vi "Main.vi"(11 "Module Admin":refnum<class "Delacor_lib_QMH_Module Admin.lvclass">) -> ()   [LabVIEW 2020, in "Logger.lvlib"]
doc: "This template is based off of the Queued Message Handler design pattern and the Queued Message Handler project template that ships with LabVIEW.\n\nThe main difference is that the queue is private to this module and communication between modules is performed via Broadcast and Request events.\n\nRequest events are wrapped in public API methods and are handled in the Event Handling Loop (EHL) of this VI. Any module can register for Broadcast events sent by this module. The EHL generates messages based on user interface actions.\n\nThe Message Handling Loop (MHL) processes messages generated by the EHL, or by other messages. The messages are string values, so new messages can be added easily to the Message Cases case structure in the MHL. Each message cluster can also provide an optional value for Message Data, which is a variant that can be converted to whatever message-specific data is required.\n_____\nBased on DQMH Project Template 4.0.0.47.\n_____\nBased on DQMH Project Template 7.0.1.1316."
uses:
  Logger.lvlib
  Module Data--cluster.ctl
  <vilib>/Delacor/Delacor QMH/Libraries/Message Queue_class/Delacor_lib_QMH_Message Queue.lvclass
  <vilib>/Delacor/Delacor QMH/Libraries/Message Queue_class/Delacor_lib_QMH_Enqueue Message (Single).vi
  <vilib>/Delacor/Delacor QMH/Libraries/Module Admin_class/Delacor_lib_QMH_Module Admin.lvclass
  Stop Argument--cluster.ctl
  <vilib>/Utility/miscctls.llb/LVPointTypeDef.ctl
  Stop Logging Argument--cluster.ctl
  Settings Editor/Settings Editor.lvlib
  Log Data Argument--cluster.ctl
  CML Shared/Signal Type--enum.ctl
  CML Shared/CML Shared.lvlib
  Settings Editor/Settings--cluster.ctl
  CML Shared/Calibration Values--cluster.ctl
  Initialize File (Reply Payload)--cluster.ctl
  Initialize File Argument--cluster.ctl
  Settings Editor/Update Application Settings (Reply Payload)--cluster.ctl
  <vilib>/Peloton/Peloton Config/DCFG Framework/Peloton_lib_DCFG Framework.lvlib
  Configuration/Configuration.lvclass
  Configuration/Configuration--cluster.ctl
  <vilib>/Peloton/Peloton Config/DCFG Framework/Configuration_class/Configuration.lvclass
panel:
  out "Settings":T1
  out "error out":errorcluster
  # "This is a headless module. Show its panel to confirm that the Settings are updated correctly and other debugging tasks. Use the Settings Editor to change the settings for this module."
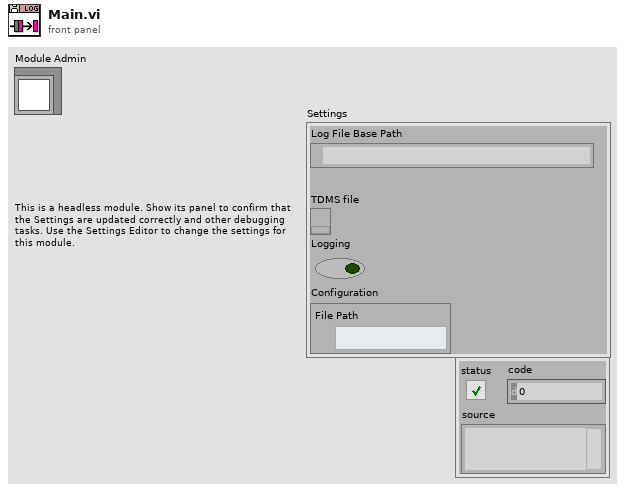
[diagram p1: front panel]
types:
  T1 = typedef "Logger.lvlib/Module Data--cluster.ctl" = cluster{"Log File Base Path":path, "TDMS file":refnum<k34>, "Logging":bool, "Configuration":T2}
  T2 = typedef "Logger.lvlib/Configuration.lvclass/Configuration--cluster.ctl" = cluster{"File Path":path}
  T3 = typedef "Settings Editor.lvlib/Broadcast Events--cluster.ctl" = cluster{"Module Did Init":refnum<user-event>, "Status Updated":refnum<user-event>, "Error Reported":refnum<user-event>, "Module Did Stop":refnum<user-event>, "Update Module Execution Status":refnum<user-event>, "Application Settings Updated":refnum<user-event>}
  T4 = typedef "Logger.lvlib/Request Events--cluster.ctl" = cluster{"Stop Module":refnum<user-event>, "Show Panel":refnum<user-event>, "Hide Panel":refnum<user-event>, "Get Module Execution Status":refnum<user-event>, "Show Diagram":refnum<user-event>, "Stop Logging":refnum<user-event>, "Log Data":refnum<user-event>, "Initialize File":refnum<user-event>}
  T5 = typedef "Peloton_lib_DCFG Framework.lvlib/Broadcast Events--cluster.ctl" = cluster{"Module Did Init":refnum<user-event>, "Status Updated":refnum<user-event>, "Error Reported":refnum<user-event>, "Module Did Stop":refnum<user-event>, "Update Module Execution Status":refnum<user-event>, "View Changed":refnum<user-event>, "Main Window Closed":refnum<user-event>, "Configuration Committed":refnum<user-event>, "Configuration Canceled":refnum<user-event>, "Views List Updated":refnum<user-event>, "Config Folder Path Updated":refnum<user-event>}
  T6 = enum32{"invalid lock state", "Not Locked", "Locked (No Password)", "Password-protected"}
  T7 = typedef "Logger.lvlib/Stop Argument--cluster.ctl" = cluster{"Origin":string, "Exit via Stop Module Req?":bool, "Wait for Module to stop?":bool}
  T8 = typedef "Logger.lvlib/Initialize File Argument--cluster.ctl" = cluster{"Wait Notifier":refnum<notifier>, "wait for reply":bool}
  T9 = typedef "Logger.lvlib/Log Data Argument--cluster.ctl" = cluster{"Waveforms":waveform(dbl)[]}
  T10 = typedef "Logger.lvlib/Stop Logging Argument--cluster.ctl" = cluster{"Boolean":bool}
  T11 = typedef "Settings Editor.lvlib/Update Application Settings (Reply Payload)--cluster.ctl" = cluster{"Settings":T12, "error":errorcluster}
  T12 = typedef "Settings Editor.lvlib/Settings--cluster.ctl" = cluster{"Signal Type":T13, "Calibration Array":T14[], "Log File Base Path":path}
  T13 = typedef "CML Shared.lvlib/Signal Type--enum.ctl" = enum16{"Sine Wave", "Square with Noise"}
  T14 = typedef "CML Shared.lvlib/Calibration Values--cluster.ctl" = cluster{"Slope":dbl, "Offset":dbl}
  T15 = typedef "LVPointTypeDef.ctl" = cluster{"Horizontal":i16, "Vertical":i16}
  T16 = enum32{"Invalid", "Standard", "Closed", "Hidden", "Minimized", "Maximized"}
  T17 = typedef "Logger.lvlib/Initialize File (Reply Payload)--cluster.ctl" = cluster{"File Path":path, "error":errorcluster}
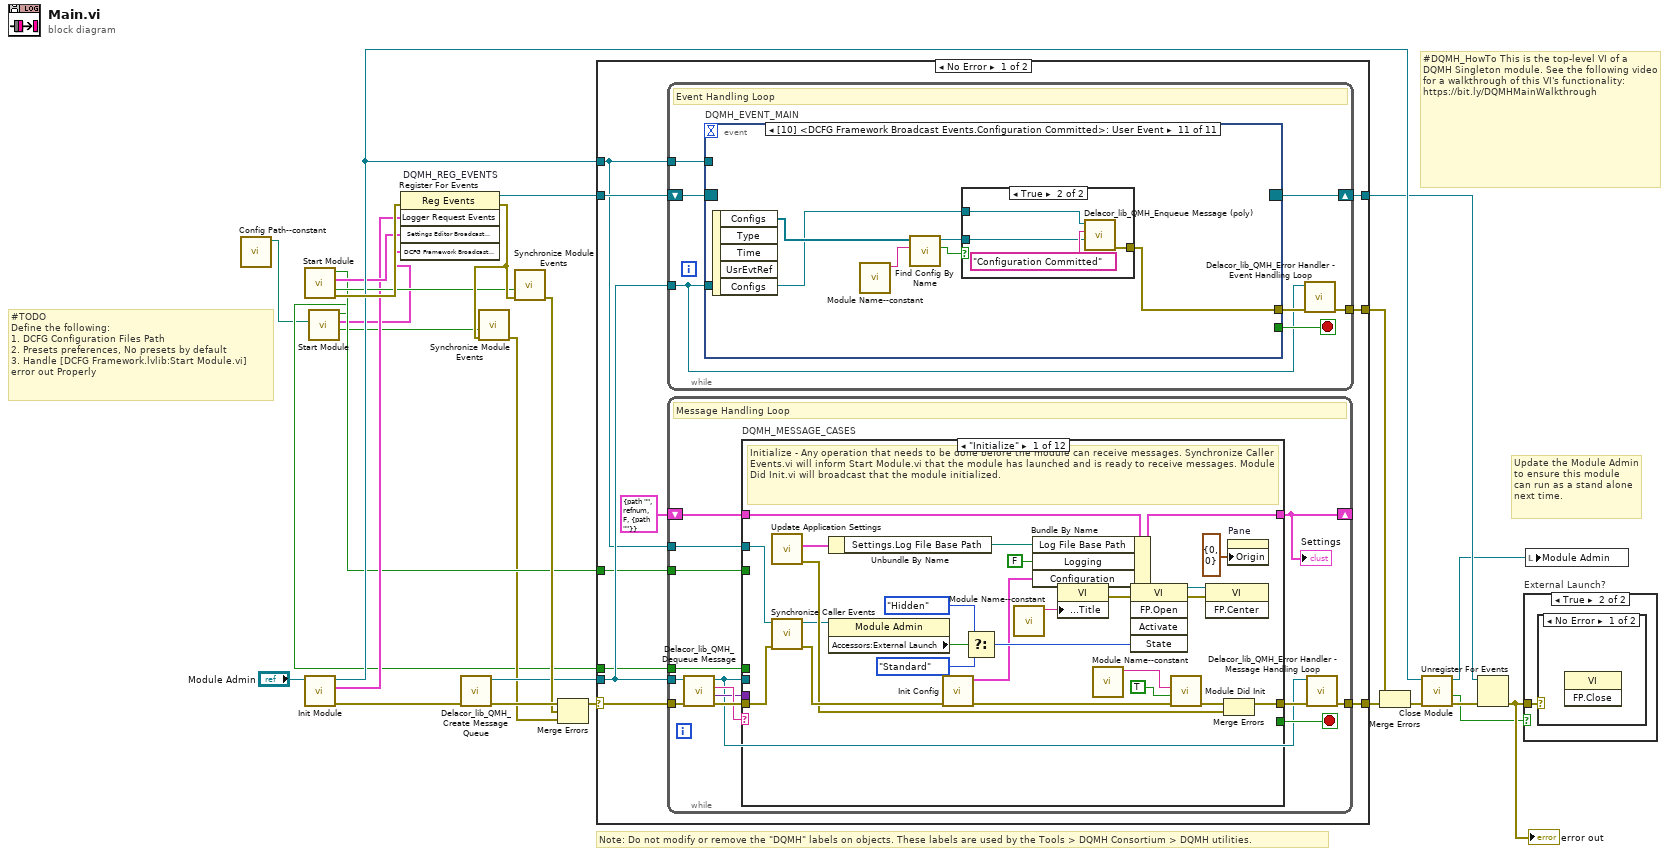
[diagram p0: block diagram]
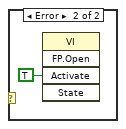
[diagram p3: hidden frame]
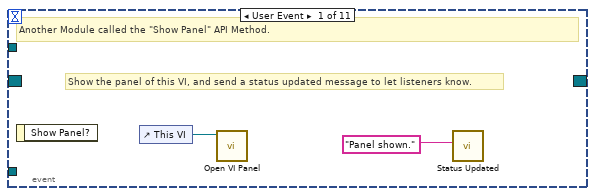
[diagram p4: hidden frame]
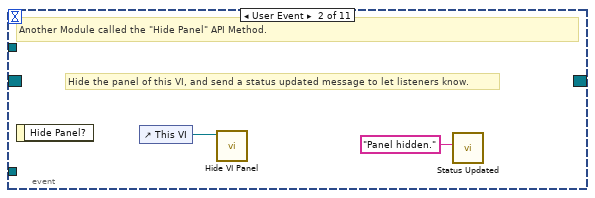
[diagram p5: hidden frame]
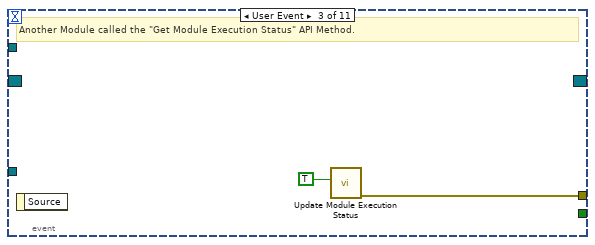
[diagram p6: hidden frame]
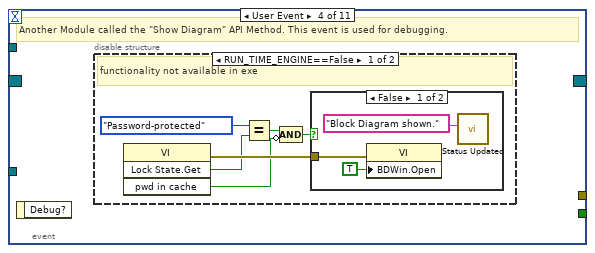
[diagram p7: hidden frame]
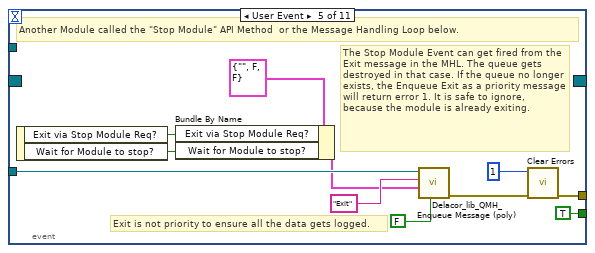
[diagram p10: hidden frame]
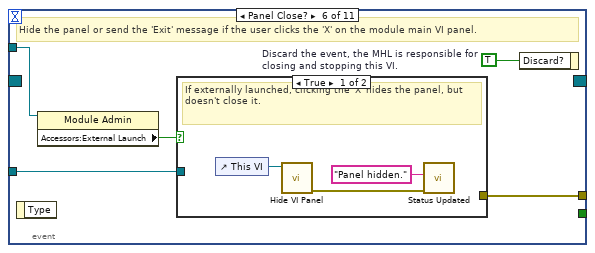
[diagram p11: hidden frame]
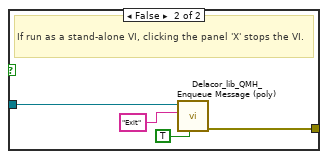
[diagram p12: hidden frame]
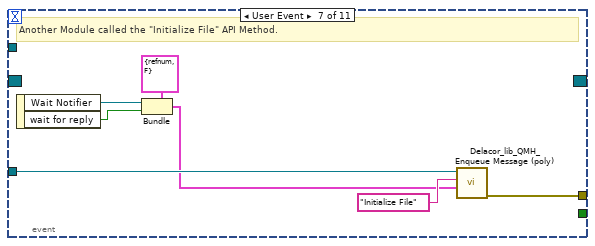
[diagram p13: hidden frame]
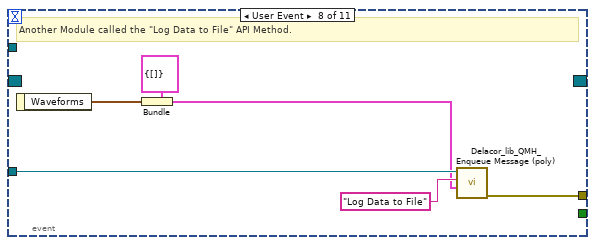
[diagram p14: hidden frame]
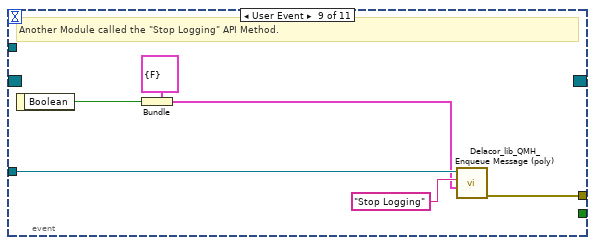
[diagram p15: hidden frame]
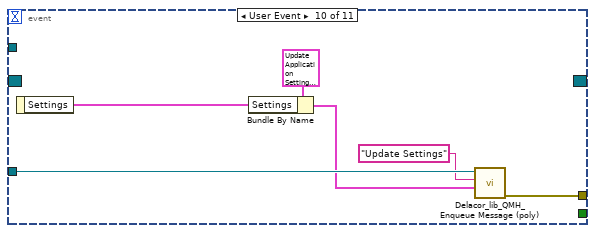
[diagram p16: hidden frame]
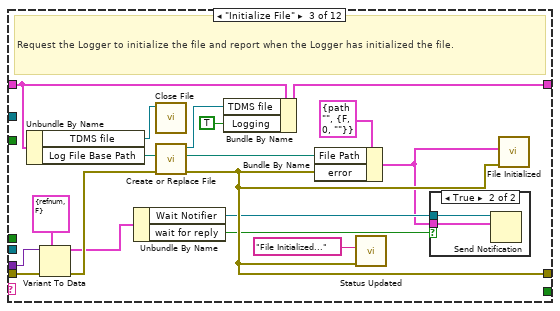
[diagram p19: hidden frame]
diagram:
  # "#TODO\nDefine the following:\n1. DCFG Configuration Files Path\n2. Presets preferences, No presets by default\n3. Handle [DCFG Framework.lvlib:Start Module.vi]\nerror out Properly"
  # "#DQMH_HowTo This is the top-level VI of a DQMH Singleton module. See the following video for a walkthrough of this VI's functionality: https://bit.ly/DQMHMainWalkthrough"
  # "Note: Do not modify or remove the \"DQMH\" labels on objects. These labels are used by the Tools > DQMH Consortium > DQMH utilities."
  # "Update the Module Admin to ensure this module can run as a stand alone next time."
  n1 = call "Config Path--constant.vi"() -> ("File Path"=w1:path)  [unwired: 11 in]
  n2 = call <vilib>:"Start Module.vi"() -> ("error out"=w19:errorcluster, "Wait for Event Sync?"=w9:bool, "Settings Editor Broadcast Events"=w8:T3, "Module Was Already Running?"=w6:bool)  [unwired: 8 in]
  n3 = call "Init Module.vi"("Singleton Module Admin in"="Module Admin") -> ("error out"=w26:errorcluster, "Logger Request Events"=w7:T4, "Singleton Module Admin out"=w16:refnum<class "Delacor_lib_QMH_Module Admin.lvclass">)  [unwired: 8 in]
  n4 = call <vilib>:"Start Module.vi"("Config Folder"=w1) -> ("Wait for Event Sync?"=w4:bool, "DCFG Framework Broadcast Events"=w5:T5, "Module Was Already Running?"=w2:bool)  [unwired: 7 in, 1 out]
  n5 = register-events "DQMH_REG_EVENTS"(error in=w19, w7, w8, w5) -> (reference out=w14:refnum<event-registration>, error out=w18:errorcluster)  [unwired: 1 in]
  n6 = call <vilib>:"Delacor_lib_QMH_Create Message Queue.vi"("error in"=w26) -> ("error out"=w21:errorcluster, "Message Queue"=w13:refnum<class "Delacor_lib_QMH_Message Queue.lvclass">)  [unwired: 9 in]
  n7 = call <vilib>:"Synchronize Module Events.vi"("error in (no error)"=w18, "Wait for Event Sync?"=w4) -> ("error out"=w3:errorcluster)  [unwired: 9 in]
  n8 = call <vilib>:"Synchronize Module Events.vi"("error in"=w18, "Wait for Event Sync?"=w9) -> ("error out"=w17:errorcluster)  [unwired: 9 in]
  n9 = Merge Errors(w21, w17, w3) -> (w20:errorcluster)
  n10 = case shown="No Error" w20 {
    selector: w20 -> [w35 w287]
    tunnel: [w37 w286] -> w27
    tunnel: [w34 w285] -> w15
    tunnel: w14 -> [w32 w285]
    tunnel: w13 -> [w31 w279]
    tunnel: [w36 _] -> w24
    tunnel: w16 -> [w30 w281]
    tunnel: w6 -> [w29 w280]
    tunnel: w2 -> [w28 w278]
    frame No Error {
      n11 = while {
        tunnel: w31 -> [w38]
        shift-right: [w41] -> w34
        shift-left: w32 -> [w42]
        tunnel: [w43] -> w36
        tunnel: w30 -> [w39]
        stop <- w40 stop-if-true
        # "Event Handling Loop"
        n12 = event "DQMH_EVENT_MAIN" shown="[10] <DCFG Framework Broadcast Events.Configuration Committed>: User Event" {
          selector: w42 -> [_ _ _ _ _ _ _ _ _ _ _]
          dyn-events: [_ _ _ _ _ _ _ _ _ _ _] -> w41
          timeout: _ -> [_ _ _ _ _ _ _ _ _ _ _]
          tunnel: [_ _ _ _ TRUE ("Discard?") _ _ _ _ _ _] -> w40
          tunnel: w38 -> [_ _ _ _ w66 w73 w88 w94 w100 w106 w111]
          tunnel: [_ _ w50 _ w69 w75 w89 w95 w101 w107 w113] -> w44
          tunnel: w39 -> [_ _ _ _ _ w72 _ _ _ _ _]
          event User Event {
            # "Show the panel of this VI, and send a status updated message to let listeners know."
            # "Another Module called the \"Show Panel\" API Method."
            n13 = event-data() -> ()  [unwired: 1 in, 1 out]
            n14 = control-ref of="This VI"() -> (w46:refnum<vi>)
            n15 = call "Open VI Panel.vi"("VI"=w46) -> ()  [unwired: 10 in, 1 out]
            n16 = call "Status Updated.vi"("Status"="Panel shown." ("format string")) -> ()  [unwired: 10 in, 1 out]
          }
          event User Event {
            # "Hide the panel of this VI, and send a status updated message to let listeners know."
            # "Another Module called the \"Hide Panel\" API Method."
            n17 = event-data() -> ()  [unwired: 1 in, 1 out]
            n18 = control-ref of="This VI"() -> (w48:refnum<vi>)
            n19 = call "Hide VI Panel.vi"("VI"=w48) -> ()  [unwired: 10 in, 1 out]
            n20 = call "Status Updated.vi"("Status"="Panel hidden." ("format string")) -> ()  [unwired: 10 in, 1 out]
          }
          event User Event {
            # "Another Module called the \"Get Module Execution Status\" API Method."
            n21 = event-data() -> ()  [unwired: 1 in, 1 out]
            n22 = call "Update Module Execution Status.vi"("Running?"=TRUE) -> ("error out"=w50:errorcluster)  [unwired: 10 in]
          }
          event User Event {
            # "Another Module called the \"Show Diagram\" API Method. This event is used for debugging."
            n23 = event-data() -> ()  [unwired: 1 in, 1 out]
            n24 = disable-structure shown="RUN_TIME_ENGINE==False" {
              frame condition #0 (active) {
                # "functionality not available in exe"
                n25 = invoke on="Invoke Node" class="VI" method="Lock State.Get"() -> (error out=w56:errorcluster, "Get Lock State"=w55:T6, "pwd in cache"=w52:bool)  [unwired: 4 in, 1 out]
                n26 = Equal?(x=T6."Password-protected", y=w55) -> (x = y?=w53:bool)
                n27 = Compound Arithmetic op=AND(w53, invert w52) -> (w51:bool)
                n28 = case shown="False" w51 {
                  tunnel: w56 -> [w59 _]
                  frame False {
                    n29 = property on="Property Node" class="VI"(error in=w59, "BDWin.Open"=TRUE ("Block Diagram Window:Open")) -> ()  [unwired: 1 in, 2 out]
                    n30 = call "Status Updated.vi"("Status"="Block Diagram shown." ("format string")) -> ()  [unwired: 10 in, 1 out]
                  }
                  frame True {
                    # "Password-protected VI, and the password is not in the cache. Do not show the diagram."
                  }
                }
              }
              frame condition #1 {
              }
            }
          }
          event User Event {
            # "Exit is not priority to ensure all the data gets logged."
            # "The Stop Module Event can get fired from the Exit message in the MHL. The queue gets destroyed in that case. If the queue no longer exists, the Enqueue Exit as a priority message will return error 1. It is safe to ignore, because the module is already exiting."
            # "Another Module called the \"Stop Module\" API Method  or the Message Handling Loop below."
            n31 = event-data() -> ("Exit via Stop Module Req?"=w62:bool, "Wait for Module to stop?"=w61:bool)  [unwired: 1 in]
            n32 = Bundle By Name(cluster=T7 {"Origin"="", "Exit via Stop Module Req?"=FALSE, "Wait for Module to stop?"=FALSE} ("Stop Argument"), "Exit via Stop Module Req?"=w62, "Wait for Module to stop?"=w61) -> (w60:T7)
            n33 = call-poly <vilib>:"Delacor_lib_QMH_Enqueue Message (poly).vi"("Priority Message? (F)"=FALSE, "Message Data"=w60, "Message"="Exit", "Message Queue in"=w66) -> ("error out"=w70:errorcluster)  [unwired: 6 in, 1 out]
            n34 = call <vilib>:"Clear Errors.vi"("error in (no error)"=w70, "specific error code to clear (0: all)"=1) -> ("error out"=w69:errorcluster)  [unwired: 4 in, 1 out]
          }
          event Panel Close? {
            w74 = TRUE  # Discard the event, the MHL is responsible for closing and stopping this VI.
            # "Hide the panel or send the 'Exit' message if the user clicks the 'X' on the module main VI panel."
            n35 = event-data() -> ()  [unwired: 1 in, 1 out]
            n36 = property on="Property Node" class="Module Admin"(reference=w72) -> ("Accessors:External Launch"=w71:bool)  [unwired: 1 in, 2 out]
            n37 = case shown="True" w71 {
              tunnel: w73 -> [_ w81]
              tunnel: [_ w82] -> w75
              frame True {
                # "If externally launched, clicking the 'X' hides the panel, but doesn't close it."
                n38 = control-ref of="This VI"() -> (w78:refnum<vi>)
                n39 = call "Hide VI Panel.vi"("VI"=w78) -> ("error out"=w76:errorcluster)  [unwired: 10 in]
                n40 = call "Status Updated.vi"("error in"=w76, "Status"="Panel hidden." ("format string")) -> ()  [unwired: 9 in, 1 out]
              }
              frame False {
                # "If run as a stand-alone VI, clicking the panel 'X' stops the VI."
                n41 = call-poly <vilib>:"Delacor_lib_QMH_Enqueue Message (poly).vi"("Priority Message? (F)"=TRUE, "Message"="Exit", "Message Queue in"=w81) -> ("error out"=w82:errorcluster)  [unwired: 7 in, 1 out]
              }
            }
            n42 = event-data ("Event Filter Node")("Discard?"=w74) -> ()  [unwired: 1 in, 1 out]
          }
          event User Event {
            # "Another Module called the \"Initialize File\" API Method."
            n43 = event-data() -> ("Wait Notifier"=w84:refnum<notifier>, "wait for reply"=w83:bool)  [unwired: 1 in]
            n44 = Bundle(cluster=T8 {"Wait Notifier"=refnum, "wait for reply"=FALSE} ("Initialize File Argument"), "Wait Notifier"=w84, "wait for reply"=w83) -> (w85:T8)
            n45 = call-poly <vilib>:"Delacor_lib_QMH_Enqueue Message (poly).vi"("Message Data"=w85, "Message"="Initialize File", "Message Queue in"=w88) -> ("error out"=w89:errorcluster)  [unwired: 7 in, 1 out]
          }
          event User Event {
            # "Another Module called the \"Log Data to File\" API Method."
            n46 = event-data() -> ("Waveforms"=w90:waveform(dbl)[])  [unwired: 1 in]
            n47 = Bundle(cluster=T9 {"Waveforms"=[]} ("Log Data to File Argument"), "Waveforms"=w90) -> (w91:T9)
            n48 = call-poly <vilib>:"Delacor_lib_QMH_Enqueue Message (poly).vi"("Message Data"=w91, "Message"="Log Data to File", "Message Queue in"=w94) -> ("error out"=w95:errorcluster)  [unwired: 7 in, 1 out]
          }
          event User Event {
            # "Another Module called the \"Stop Logging\" API Method."
            n49 = event-data() -> ("Boolean"=w96:bool)  [unwired: 1 in]
            n50 = Bundle(cluster=T10 {"Boolean"=FALSE} ("Stop Logging Argument"), "Boolean"=w96) -> (w97:T10)
            n51 = call-poly <vilib>:"Delacor_lib_QMH_Enqueue Message (poly).vi"("Message Data"=w97, "Message"="Stop Logging", "Message Queue in"=w100) -> ("error out"=w101:errorcluster)  [unwired: 7 in, 1 out]
          }
          event User Event {
            n52 = event-data() -> ("Settings"=w103:T12)  [unwired: 1 in]
            n53 = Bundle By Name(cluster=T11 {"Settings"={"Signal Type"=enum."Sine Wave", "Calibration Array"=[], "Log File Base Path"=path ""}, "error"={"status"=FALSE, "code"=0, "source"=""}} ("Settings Updated Argument"), "Settings"=w103) -> (w102:T11)
            n54 = call-poly <vilib>:"Delacor_lib_QMH_Enqueue Message (poly).vi"("Message Data"=w102, "Message"="Update Settings", "Message Queue in"=w106) -> ("error out"=w107:errorcluster)  [unwired: 7 in, 1 out]
          }
          event User Event {
            n55 = event-data() -> ("Configs"=w112:refnum<class "Configuration.lvclass">[])  [unwired: 1 in, 4 out]
            n56 = call "Module Name--constant.vi"() -> ("Module Name"=w110:string)  [unwired: 11 in]
            n57 = call <vilib>:"Find Config By Name.vi"("Config Name"=w110, "All Config Classes"=w112) -> ("Found"=w109:bool, "Configuration"=w108:refnum<class "Configuration.lvclass">)  [unwired: 6 in, 2 out]
            n58 = case shown="True" w109 {
              tunnel: w111 -> [_ w116]
              tunnel: [_ w117] -> w113
              tunnel: w108 -> [_ w114]
              frame False {
              }
              frame True {
                n59 = call-poly <vilib>:"Delacor_lib_QMH_Enqueue Message (poly).vi"("Message Data"=w114, "Message"="Configuration Committed", "Message Queue in"=w116) -> ("error out"=w117:errorcluster)  [unwired: 7 in, 1 out]
              }
            }
          }
        }
        n60 = call-dynamic "Delacor_lib_QMH_Error Handler - Event Handling Loop.vi"("error in"=w44, "Message Queue in"=w38) -> ("dup error in"=w43:errorcluster)  [unwired: 8 in, 1 out]
      }
      n61 = while {
        tunnel: w31 -> [w122]
        shift-right: [w126] -> _
        shift-left: T1 {"Log File Base Path"=path "", "TDMS file"=refnum, "Logging"=FALSE, "Configuration"={"File Path"=path ""}} ("Data Cluster") -> [w127]
        tunnel: w35 -> [w130]
        tunnel: [w128] -> w37
        tunnel: w30 -> [w120]
        tunnel: w29 -> [w119]
        tunnel: w28 -> [w118]
        stop <- w125 stop-if-true
        # "Message Handling Loop"
        n62 = call-dynamic "Delacor_lib_QMH_Dequeue Message.vi"("error in"=w130, "Message Queue in"=w122) -> ("error out"=w129:errorcluster, "Message Data"=w123:variant, "Message"=w124:string, "Message Queue out"=w121:refnum<class "Delacor_lib_QMH_Message Queue.lvclass">)  [unwired: 6 in]
        n63 = case "DQMH_MESSAGE_CASES" shown="\"Initialize\"" w124 {
          selector: w124 -> [_ _ _ _ _ _ _ _ _ _ w265 _]
          tunnel: w121 -> [_ _ _ _ _ _ _ _ w225 w251 _ _]
          tunnel: w129 -> [w155 w159 w176 w188 w201 w211 w219 w221 w232 w257 w268 w277]
          tunnel: [w152 w159 w177 w187 w200 w209 w218 w221 w228 w252 w269 w274] -> w131
          tunnel: w127 -> [w142 w158 w165 w184 w199 w204 w217 w220 w227 w243 w266 w276]
          tunnel: [w136 w158 w164 w181 w197 w204 w217 w220 w227 w243 w266 w275] -> w126
          tunnel: [_ _ _ _ _ _ _ _ _ w250 _ _] -> w125
          tunnel: w123 -> [_ _ w174 w186 w198 w208 _ _ w226 w249 _ w273]
          tunnel: w120 -> [w143 _ _ _ _ _ _ _ w224 w244 _ _]
          tunnel: w119 -> [_ _ _ _ _ _ _ _ _ w241 _ _]
          tunnel: w118 -> [_ _ _ _ _ _ _ _ _ w239 _ _]
          frame "Initialize" {
            # "Initialize - Any operation that needs to be done before the module can receive messages. Synchronize Caller Events.vi will inform Start Module.vi that the module has launched and is ready to receive messages. Module Did Init.vi will broadcast that the module initialized."
            n64 = call "Update Application Settings.vi"() -> ("error out"=w151:errorcluster, "Reply Payload"=w137:T11)  [unwired: 9 in, 1 out]
            n65 = call "Synchronize Caller Events.vi"("error in"=w155, "Singleton Module Admin in"=w143) -> ("error out"=w154:errorcluster, "Singleton Module Admin out"=w139:refnum<class "Delacor_lib_QMH_Module Admin.lvclass">)  [unwired: 8 in]
            n66 = Unbundle By Name(w137) -> ("Settings.Log File Base Path"=w135:path)
            n67 = property on="Property Node" class="Module Admin"(reference=w139) -> ("Accessors:External Launch"=w147:bool)  [unwired: 1 in, 2 out]
            n68 = call "Init Config.vi"("error in"=w154) -> ("error out"=w133:errorcluster, "Configuration"=w132:T2)  [unwired: 9 in]
            n69 = Select(t=T16."Hidden" ("State"), s=w147, f=T16."Standard" ("State")) -> (s? t:f=w144:T16)
            n70 = call "Module Name--constant.vi"() -> ("Module Name"=w150:string)  [unwired: 11 in]
            n71 = Bundle By Name(cluster=w142, "Log File Base Path"=w135, "Logging"=FALSE, "Configuration"=w132) -> (w136:T1)
            n72 = property on="Property Node" class="VI"("Front Panel.Title"=w150) -> (reference out=w149:refnum<vi>, error out=w157:errorcluster)  [unwired: 2 in]
            n73 = call "Module Name--constant.vi"() -> ("Module Name"=w140:string)  [unwired: 11 in]
            n74 = invoke on="Invoke Node" class="VI" method="FP.Open"(reference=w149, error in=w157, "State"=w144) -> (reference out=w148:refnum<vi>, error out=w156:errorcluster)  [unwired: 2 in, 3 out]
            n75 = call "Module Did Init.vi"("error in"=w133, "Initialized?"=TRUE, "Origin"=w140) -> ("error out"=w153:errorcluster)  [unwired: 8 in]
            n76 = invoke on="Invoke Node" class="VI" method="FP.Center"(reference=w148, error in=w156) -> ()  [unwired: 1 in, 3 out]
            n77 = Merge Errors(w153, w151) -> (w152:errorcluster)
            n78 = property on="Pane" class="Pane"("Origin"=T15 {"Horizontal"=0, "Vertical"=0}) -> ()  [unwired: 2 in, 2 out]
          }
          frame "---Module Specific---" {
            # "Separator -- The following cases handle messages specific to this Module."
          }
          frame "Initialize File" {
            # "Request the Logger to initialize the file and report when the Logger has initialized the file."
            n79 = Unbundle By Name(w165) -> ("TDMS file"=w160:refnum<k34>, "Log File Base Path"=w167:path)
            n80 = Variant To Data(error in=w176, type=T8 {"Wait Notifier"=refnum, "wait for reply"=FALSE} ("Initialize File Argument"), Variant=w174) -> (data=w172:T8, error out=w175:errorcluster)
            n81 = Unbundle By Name(w172) -> ("Wait Notifier"=w171:refnum<notifier>, "wait for reply"=w170:bool)
            n82 = call "Close File.vi"("Refnum out"=w160) -> ()  [unwired: 10 in, 1 out]
            n83 = call "Create or Replace File.vi"("error in"=w175, "Log File Base Path"=w167) -> ("error out"=w177:errorcluster, "File Path"=w163:path, "Refnum out"=w166:refnum<k34>)  [unwired: 7 in]
            n84 = Bundle By Name(cluster=w165, "TDMS file"=w166, "Logging"=TRUE) -> (w164:T1)
            n85 = Bundle By Name(cluster=T17 {"File Path"=path "", "error"={"status"=FALSE, "code"=0, "source"=""}} ("Initialize File (Reply Payload)"), "File Path"=w163, "error"=w177) -> (w168:T17)
            n86 = call "Status Updated.vi"("error in"=w177, "Status"="File Initialized...") -> ()  [unwired: 9 in, 1 out]
            n87 = case shown="True" w170 {
              tunnel: w171 -> [_ w179]
              tunnel: w168 -> [_ w178]
              frame False {
              }
              frame True {
                n88 = Send Notification(notification=w178, notifier=w179) -> ()  [unwired: 1 in, 2 out]
              }
            }
            n89 = call "File Initialized.vi"("error in"=w177, "Reply Payload"=w168) -> ()  [unwired: 9 in, 1 out]
          }
          frame "Stop Logging" {
            # "Requests Logger module to stop logging and the module broadcasts when the logging has stopped."
            n90 = Variant To Data(error in=w188, type=T10 {"Boolean"=FALSE} ("Stop Logging Argument"), Variant=w186) -> (error out=w187:errorcluster)  [unwired: 1 out]
            n91 = Unbundle By Name(w184) -> ("Logging"=w183:bool, "TDMS file"=w182:refnum<k34>)
            n92 = case shown="True" w183 {
              tunnel: w187 -> [_ w192]
              tunnel: w182 -> [_ w189]
              frame False {
                # "We were not logging, so this is a no-op."
              }
              frame True {
                n93 = call "Close File.vi"("Refnum out"=w189) -> ()  [unwired: 10 in, 1 out]
                n94 = call "Logging Stopped.vi"("error in"=w192) -> ("error out"=w191:errorcluster)  [unwired: 10 in]
                n95 = call "Status Updated.vi"("error in"=w191, "Status"="Logging Stopped...") -> ()  [unwired: 9 in, 1 out]
              }
            }
            n96 = Bundle By Name(cluster=w184, "Logging"=FALSE) -> (w181:T1)
          }
          frame "Update Settings" {
            n97 = Variant To Data(error in=w201, type=T11 {"Settings"={"Signal Type"=enum."Sine Wave", "Calibration Array"=[], "Log File Base Path"=path ""}, "error"={"status"=FALSE, "code"=0, "source"=""}} ("Settings Updated Argument"), Variant=w198) -> (data=w196:T11, error out=w200:errorcluster)
            n98 = Unbundle By Name(w196) -> ("Settings.Log File Base Path"=w195:path)
            n99 = Bundle By Name(cluster=w199, "Log File Base Path"=w195) -> (w197:T1)
            n100 = call "Status Updated.vi"("error in"=w200, "Status"="Settings Updated") -> ()  [unwired: 9 in, 1 out]
          }
          frame "Log Data to File" {
            # "Requests Logger module to log data to file"
            n101 = Variant To Data(error in=w211, type=T9 {"Waveforms"=[]} ("Log Data to File Argument"), Variant=w208) -> (data=w206:T9, error out=w210:errorcluster)
            n102 = Unbundle By Name(w204) -> ("Logging"=w202:bool, "TDMS file"=w203:refnum<k34>)
            n103 = Unbundle By Name(w206) -> ("Waveforms"=w205:waveform(dbl)[])
            n104 = case shown="True" w202 {
              tunnel: w210 -> [w212 w216]
              tunnel: [w212 w215] -> w209
              tunnel: w205 -> [_ w214]
              tunnel: w203 -> [_ w213]
              frame False {
                # "We are not currently logging, so this action is a no-op."
              }
              frame True {
                n105 = call "Log Data to File.vi"("error in"=w216, "Data to log"=w214, "TDMS File Reference"=w213) -> ("error out"=w215:errorcluster)  [unwired: 8 in]
              }
            }
          }
          frame "---Copy This Frame---" {
            # "Duplicate this frame when creating new messages.  Change this comment in the duplicated frame to describe this message."
            n106 = Merge Errors(w219) -> (w218:errorcluster)
          }
          frame "---Exit and Error Handling---" {
            # "Separator - The following cases handle errors and exit messages."
          }
          frame "Error" {
            # "Error - Check the error message data and respond accordingly. This message is sent by the \"Error Handler\" VIs at the end of each loop in this application."
            n107 = property on="Property Node" class="Module Admin"(reference=w224) -> ("Accessors:External Launch"=w223:bool)  [unwired: 1 in, 2 out]
            n108 = Variant To Data(error in=w232, type=errorcluster {"status"=FALSE, "code"=0, "source"=""} ("error constant"), Variant=w226) -> (data=w222:errorcluster, error out=w230:errorcluster)
            n109 = local write "error out"(w222) -> ()
            n110 = call "Error Reported.vi"("Error"=w222) -> ()  [unwired: 10 in, 1 out]
            n111 = case shown="False" w223 {
              tunnel: [w237 _] -> w229
              tunnel: w225 -> [w235 _]
              tunnel: w222 -> [w236 _]
              frame False {
                n112 = disable-structure shown="Default" {
                  disable-tunnel: w236 -> [w238 _]
                  frame condition #0 (active) {
                    # "If the module is running standalone, then pop up an error dialog and call the \"Exit\" message."
                    n113 = call <vilib>:"Simple Error Handler.vi"("error in (no error)"=w238) -> ()  [unwired: 4 in, 5 out]
                  }
                  frame condition #1 {
                    # "To prevent the Simple Error Handler VI from being loaded (e.g. when deploying to a Real-Time target), add the Conditional Disable Symbol \"DQMH_Disable_SEH\" to your project and set it to TRUE."
                  }
                }
                n114 = call-poly <vilib>:"Delacor_lib_QMH_Enqueue Message (poly).vi"("Priority Message? (F)"=TRUE, "Message"="Exit", "Message Queue in"=w235) -> ("error out"=w237:errorcluster)  [unwired: 7 in, 1 out]
              }
              frame True {
                # "If the module was launched externally, calling the Error Reported broadcast VI is the only action performed by the \"Error\" message. The module's caller can then process the error appropriately."
              }
            }
            n115 = Merge Errors(w230, w229) -> (w228:errorcluster)
          }
          frame "Exit" {
            w250 = TRUE  # Stop the VI
            # "Release the message queue reference"
            # "Exit - Exit the application."
            n116 = Variant To Data(error in=w257, type=T7 {"Origin"="", "Exit via Stop Module Req?"=FALSE, "Wait for Module to stop?"=FALSE} ("Stop Argument"), Variant=w249) -> (data=w246:T7, error out=w254:errorcluster)
            n117 = call <vilib>:"Clear Errors.vi"("error in (no error)"=w254, "specific error code to clear (0: all)"=91 ("91: not all Exit messages will have an argument")) -> ("error out"=w256:errorcluster)  [unwired: 4 in, 1 out]
            n118 = Unbundle By Name(w243) -> ("TDMS file"=w242:refnum<k34>)
            n119 = control-ref of="This VI"() -> (w245:refnum<vi>)
            n120 = call-dynamic "Delacor_lib_QMH_Release Message Queue.vi"("error in"=w256, "Message Queue"=w251) -> ("error out"=w255:errorcluster)  [unwired: 9 in]
            n121 = call "Handle Exit.vi"("Stop Argument"=w246, "Admin in"=w244, "VI reference"=w245) -> ("error out"=w253:errorcluster)  [unwired: 7 in, 1 out]
            n122 = call "Close File.vi"("Refnum out"=w242) -> ()  [unwired: 10 in, 1 out]
            n123 = call "Destroy Config.vi"() -> ("error out"=w240:errorcluster)  [unwired: 11 in]
            n124 = case "DCFG_Stop_Case" shown="False" w239 {
              tunnel: w240 -> [_ _]
              frame False {
                n125 = call <vilib>:"Stop Module.vi"() -> ()  [unwired: 11 in, 1 out]
              }
              frame True {
                # "Let DCFG Running if it was already running"
              }
            }
            n126 = case "Settings Editor was\nalready running?" shown="False" w241 {
              frame False {
                n127 = call "Module Name--constant.vi"() -> ("Module Name"=w259:string)  [unwired: 11 in]
                n128 = call <vilib>:"Stop Module.vi"("Wait for Module to Stop? (F)"=TRUE, "Origin"=w259) -> ()  [unwired: 9 in, 1 out]
              }
              frame True {
                # "Another Module is\nin charge of stopping Settings Editor"
              }
            }
            n129 = Merge Errors(w255, w253) -> (w252:errorcluster)
            n130 = call "Error Reported.vi"("Error"=w252) -> ()  [unwired: 10 in, 1 out]
          }
          frame Default {
            # "'Default' case only runs if there is a message that isn't defined in any of the other cases.  Output a programming error."
            n131 = call "Module Name--constant.vi"() -> ("Module Name"=w264:string)  [unwired: 11 in]
            n132 = Format Into String(format string="The invalid message string \"%s\" was received in the Message Handling Loop for module \"%s\".", w265, w264) -> (resulting string=w262:string)  [unwired: 2 in, 1 out]
            n133 = call <vilib>:"Error Cluster From Error Code.vi"("show call chain? (False)"=TRUE, "error message (\"\")"=w262, "error code (0)"=1) -> ("error out"=w267:errorcluster)  [unwired: 6 in]
            n134 = Merge Errors(w268, w267) -> (w269:errorcluster)
          }
          frame "Configuration Committed" {
            w271 = refnum<class "Configuration.lvclass"> refnum  # Module_Config_Class
            n135 = Variant To Data(error in=w277, type=w271, Variant=w273) -> (data=w270:refnum<class "Configuration.lvclass">, error out=w274:errorcluster)
            n136 = property on="Property Node" class="Config"(reference=w270) -> ("Accessors:Configuration"=w272:T2)  [unwired: 1 in, 2 out]
            n137 = Bundle By Name(cluster=w276, "Configuration"=w272) -> (w275:T1)
          }
        }
        "Settings" <- w126
        n138 = call-dynamic "Delacor_lib_QMH_Error Handler - Message Handling Loop.vi"("error in"=w131, "Message Queue in"=w121) -> ("dup error in"=w128:errorcluster)  [unwired: 8 in, 1 out]
      }
    }
    frame Error {
      # "Synchronize Caller Events.vi will inform Start Module.vi that the module has launched and will let the code calling Start Module.vi register for broadcasts and would permit the caller receive the broadcast that an error occurred at launch time."
      n139 = call "Synchronize Caller Events.vi"("Singleton Module Admin in"=w281) -> ("error out"=w288:errorcluster)  [unwired: 9 in, 1 out]
      n140 = call-dynamic "Delacor_lib_QMH_Release Message Queue.vi"("error in"=w287, "Message Queue"=w279) -> ("error out"=w286:errorcluster)  [unwired: 9 in]
      n141 = call "Module Name--constant.vi"() -> ("Module Name"=w284:string)  [unwired: 11 in]
      n142 = case "Settings Editor was\nalready running?" shown="False" w280 {
        frame False {
          n143 = call "Module Name--constant.vi"() -> ("Module Name"=w291:string)  [unwired: 11 in]
          n144 = call <vilib>:"Stop Module.vi"("Wait for Module to Stop? (F)"=TRUE, "Origin"=w291) -> ()  [unwired: 9 in, 1 out]
        }
        frame True {
          # "Another Module is\nin charge of stopping Settings Editor"
        }
      }
      n145 = Format Into String(format string="An error occurred during initialization. %s is no longer running.", w284) -> (resulting string=w282:string)  [unwired: 2 in, 1 out]
      n146 = Merge Errors(w287, w288) -> (w289:errorcluster)
      n147 = case "DCFG_Stop_Case" shown="False" w278 {
        frame False {
          n148 = call <vilib>:"Stop Module.vi"() -> ()  [unwired: 11 in, 1 out]
        }
        frame True {
          # "Let DCFG Running if it was already running"
        }
      }
      n149 = call "Error Reported.vi"("Additional Information"=w282, "Error"=w289) -> ()  [unwired: 9 in, 1 out]
    }
  }
  n150 = Merge Errors(w24, w27) -> (w23:errorcluster)
  n151 = call "Close Module.vi"("error in"=w23, "Module Admin in"=w16) -> ("error out"=w25:errorcluster, "External Launch"=w10:bool, "Module Admin out"=w11:refnum<class "Delacor_lib_QMH_Module Admin.lvclass">)  [unwired: 7 in]
  n152 = Unregister For Events(event registration refnum=w15, error in=w25) -> (error out=w22:errorcluster)
  "error out" <- w22
  n153 = case "External Launch?" shown="True" w10 {
    tunnel: w22 -> [_ w292]
    frame False {
    }
    frame True {
      n154 = case shown="No Error" w292 {
        frame No Error {
          n155 = invoke on="Invoke Node" class="VI" method="FP.Close"() -> ()  [unwired: 3 in, 3 out]
        }
        frame Error {
          n156 = invoke on="Invoke Node" class="VI" method="FP.Open"("Activate"=TRUE ("Activate?")) -> ()  [unwired: 4 in, 5 out]
        }
      }
    }
  }
  n157 = local write "Module Admin"(w11) -> ()
